vi "BRig_Host_dataRunState__dataPlot_idxANDcol_get.vi"(10 "input_tSelection_plot":u16, 11 "input_sSelection":u16) -> (2 "output_col_dataPlot":i32, 3 "output_idx_dataPlot":i32)   [LabVIEW 2014]
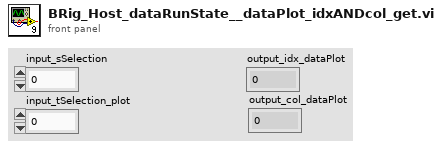
[diagram p1: front panel]
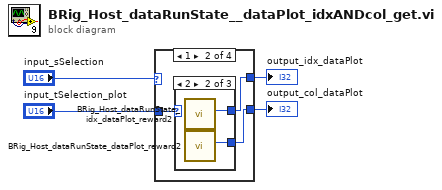
[diagram p0: block diagram]
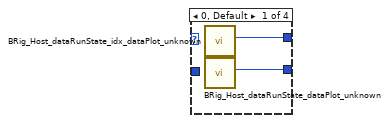
[diagram p2: hidden frame]
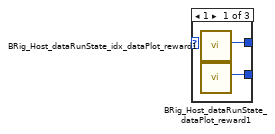
[diagram p3: hidden frame]
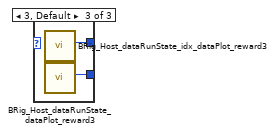
[diagram p4: hidden frame]
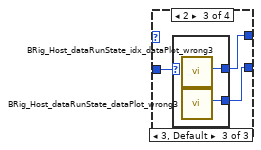
[diagram p5: hidden frame]
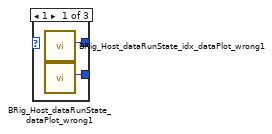
[diagram p6: hidden frame]
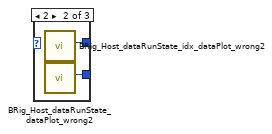
[diagram p7: hidden frame]
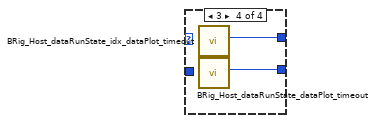
[diagram p8: hidden frame]
diagram:
  n1 = case shown="1" "input_sSelection" {
    tunnel: [w6 w8 w17 w26] -> w2
    tunnel: "input_tSelection_plot" -> [_ w9 w18 _]
    tunnel: [w5 w7 w16 w25] -> w1
    frame 0, Default {
      n2 = call "BRig_Host_dataRunState_idx_dataPlot_unknown.vi"() -> ("output_idx_dataPlot_unknown"=w6:i32)  [unwired: 11 in]
      n3 = call "BRig_Host_dataRunState_dataPlot_unknown.vi"() -> ("output_idx_dataPlot_unknown"=w5:i32)  [unwired: 11 in]
    }
    frame 1 {
      n4 = case shown="2" w9 {
        tunnel: [w11 w13 w15] -> w8
        tunnel: [w10 w12 w14] -> w7
        frame 1 {
          n5 = call "BRig_Host_dataRunState_idx_dataPlot_reward1.vi"() -> ("output_idx_dataPlot_reward1"=w11:i32)  [unwired: 11 in]
          n6 = call "BRig_Host_dataRunState_dataPlot_reward1.vi"() -> ("output_idx_dataPlot_reward1"=w10:i32)  [unwired: 11 in]
        }
        frame 2 {
          n7 = call "BRig_Host_dataRunState_idx_dataPlot_reward2.vi"() -> ("output_idx_dataPlot_reward2"=w13:i32)  [unwired: 11 in]
          n8 = call "BRig_Host_dataRunState_dataPlot_reward2.vi"() -> ("output_idx_dataPlot_reward2"=w12:i32)  [unwired: 11 in]
        }
        frame 3, Default {
          n9 = call "BRig_Host_dataRunState_idx_dataPlot_reward3.vi"() -> ("output_idx_dataPlot_reward3"=w15:i32)  [unwired: 11 in]
          n10 = call "BRig_Host_dataRunState_dataPlot_reward3.vi"() -> ("output_idx_dataPlot_reward3"=w14:i32)  [unwired: 11 in]
        }
      }
    }
    frame 2 {
      n11 = case shown="3, Default" w18 {
        tunnel: [w20 w22 w24] -> w17
        tunnel: [w19 w21 w23] -> w16
        frame 1 {
          n12 = call "BRig_Host_dataRunState_idx_dataPlot_wrong1.vi"() -> ("output_idx_dataPlot_wrong1"=w20:i32)  [unwired: 11 in]
          n13 = call "BRig_Host_dataRunState_dataPlot_wrong1.vi"() -> ("output_idx_dataPlot_wrong1"=w19:i32)  [unwired: 11 in]
        }
        frame 2 {
          n14 = call "BRig_Host_dataRunState_idx_dataPlot_wrong2.vi"() -> ("output_idx_dataPlot_wrong2"=w22:i32)  [unwired: 11 in]
          n15 = call "BRig_Host_dataRunState_dataPlot_wrong2.vi"() -> ("output_idx_dataPlot_wrong2"=w21:i32)  [unwired: 11 in]
        }
        frame 3, Default {
          n16 = call "BRig_Host_dataRunState_idx_dataPlot_wrong3.vi"() -> ("output_idx_dataPlot_wrong3"=w24:i32)  [unwired: 11 in]
          n17 = call "BRig_Host_dataRunState_dataPlot_wrong3.vi"() -> ("output_idx_dataPlot_wrong3"=w23:i32)  [unwired: 11 in]
        }
      }
    }
    frame 3 {
      n18 = call "BRig_Host_dataRunState_idx_dataPlot_timeout.vi"() -> ("output_idx_dataPlot_timeout"=w26:i32)  [unwired: 11 in]
      n19 = call "BRig_Host_dataRunState_dataPlot_timeout.vi"() -> ("output_idx_dataPlot_timeout"=w25:i32)  [unwired: 11 in]
    }
  }
  "output_idx_dataPlot" <- w2
  "output_col_dataPlot" <- w1
